vi "Set-KeyValue-Section.vi"(6 "Value":string, 8 "error in (no error)":errorcluster, 9 "Key":string, 10 "Section":string, 11 "Config in":refnum<class "Config.lvclass">) -> (0 "error out":errorcluster, 3 "Config out":refnum<class "Config.lvclass">)   [LabVIEW 2020, in "Config.lvclass"]
uses:
  Config.lvclass
  <userlib>/_OpenG.lib/dictionary/dictionary.llb/Dictionary Object RefNum__ogtk.ctl
  <userlib>/_OpenG.lib/dictionary/dictionary.llb/Dictionary Object RefNum - Enum__ogtk.ctl
  Config.lvclass/Config.ctl
  <userlib>/_OpenG.lib/dictionary/dictionary.llb/Dictionary Update (by scalar value)__ogtk.vi
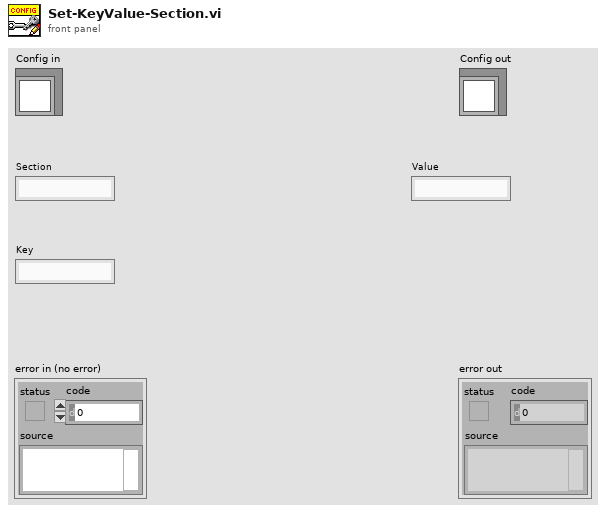
[diagram p1: front panel]
types:
  T1 = typedef "Dictionary Object RefNum__ogtk.ctl" = refnum<k1>
  T2 = cluster{"Keys":string[], "Keys-values":string[]}[]
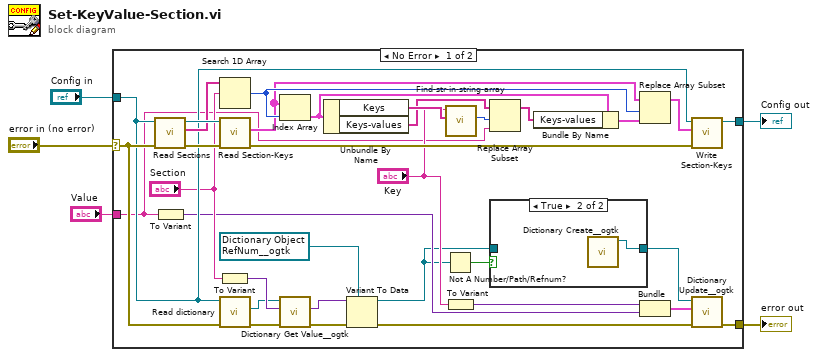
[diagram p0: block diagram]
diagram:
  n1 = case shown="No Error" "error in (no error)" {
    selector: "error in (no error)" -> [w24 w42]
    tunnel: [w9 w42] -> w4
    tunnel: [w30 w41] -> w2
    tunnel: "Config in" -> [w23 w41]
    tunnel: "Value" -> [w13 _]
    frame No Error {
      w17 = T1 refnum items=["Dictionary"] ("Object RefNum")
      n2 = call "Read Sections.vi"("error in (no error)"=w24, "Config in"=w23) -> ("error out"=w37:errorcluster, "Sections"=w35:string[], "Config out"=w38:refnum<class "Config.lvclass">)  [unwired: 7 in]
      n3 = To Variant(anything=w13) -> (Variant=w12:variant)
      n4 = Search 1D Array(1D array=w35, element="Section") -> (index of element=w28:i32)  [unwired: 1 in]
      n5 = call "Read Section-Keys.vi"("error in (no error)"=w37, "Config in"=w38) -> ("error out"=w29:errorcluster, "Section-Keys"=w27:T2)  [unwired: 7 in, 1 out]
      n6 = To Variant(anything="Section") -> (Variant=w20:variant)
      n7 = call "Read dictionary.vi"("error in (no error)"=w24, "Config in"=w23) -> ("error out"=w21:errorcluster, "Object RefNum"=w19:T1)  [unwired: 7 in, 1 out]
      n8 = Index Array(array=w27, index=w28) -> (element=w32:cluster{"Keys":string[], "Keys-values":string[]})
      n9 = call <userlib>:"Dictionary Get Value__ogtk.vi"("error in"=w21, "key"=w20, "dictionary"=w19) -> ("error out"=w16:errorcluster, "value"=w18:variant)  [unwired: 5 in, 2 out]
      n10 = Unbundle By Name(w32) -> ("Keys"=w36:string[], "Keys-values"=w34:string[])
      n11 = Variant To Data(error in=w16, type=w17, Variant=w18) -> (data=w6:T1, error out=w15:errorcluster)
      n12 = Not A Number/Path/Refnum?(number/path/refnum=w6) -> (NaN/Path/Refnum?=w8:bool)
      n13 = call "Find-str-in-string-array.vi"("str array"=w36, "str"="Key") -> ("found index"=w33:i32)  [unwired: 9 in]
      n14 = To Variant(anything="Key") -> (Variant=w11:variant)
      n15 = Replace Array Subset(array=w34, new element=w13, index=w33) -> (w31:string[])
      n16 = case shown="True" w8 {
        tunnel: [w39 w40] -> w7
        tunnel: w6 -> [w39 _]
        frame False {
        }
        frame True {
          n17 = call <userlib>:"Dictionary Create__ogtk.vi"() -> ("dictionary out"=w40:T1)  [unwired: 10 in, 1 out]
        }
      }
      n18 = Bundle By Name(cluster=w32, "Keys-values"=w31) -> (w26:cluster{"Keys":string[], "Keys-values":string[]})
      n19 = Replace Array Subset(array=w27, new element=w26, index=w28) -> (w25:T2)
      n20 = Bundle("Variant"=w11, "Variant"=w12) -> (w10:cluster{"Variant":variant, "Variant":variant})  [unwired: 1 in]
      n21 = call "Write Section-Keys.vi"("error in (no error)"=w29, "Section-Keys"=w25, "Config in"=w23) -> ("Config out"=w30:refnum<class "Config.lvclass">)  [unwired: 7 in, 1 out]
      n22 = call-poly <userlib>:"Dictionary Update__ogtk.vi"("error in (no error)"=w15, "key-value"=w10, "dictionary"=w7) -> ("error out"=w9:errorcluster)  [unwired: 6 in, 2 out]
    }
    frame Error {
    }
  }
  "error out" <- w4
  "Config out" <- w2
